vi "Pos ctrl window-Update coord indicators.vi"(9 "Z":sgl, 10 "Y":sgl, 11 "X":sgl) -> ()   [LabVIEW 2020]
uses:
  Globals/Pos ctrl window globals.vi
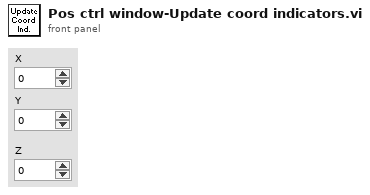
[diagram p1: front panel]
types:
  T1 = typedef "Pos Ctrl window refs cluster.ctl" = cluster{"menu reference":refnum<k9>, "X Coordinate ctrl":refnum<vi>, "Y Coordinate ctrl":refnum<vi>, "Z Coordinate ctrl":refnum<vi>, "Speed setting ctrl":refnum<vi>, "Up":refnum<vi>, "Down":refnum<vi>, "Left":refnum<vi>, "Right":refnum<vi>, "Z move up":refnum<vi>, "Z move down":refnum<vi>, "Down-left":refnum<vi>, "Down-right":refnum<vi>, "Up-left":refnum<vi>, "Up-right":refnum<vi>, "Step = size of image":refnum<vi>, "XY step (um)":refnum<vi>, "Z step (um)":refnum<vi>}
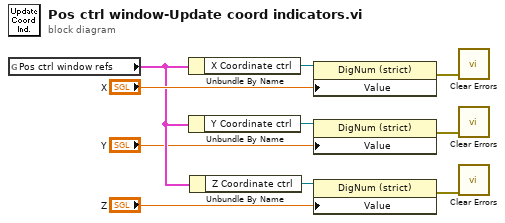
[diagram p0: block diagram]
diagram:
  n1 = global read "Pos ctrl window globals.vi" "Pos ctrl window refs"() -> (w2:T1)
  n2 = Unbundle By Name(w2) -> ("X Coordinate ctrl"=w10:refnum<vi>)
  n3 = Unbundle By Name(w2) -> ("Y Coordinate ctrl"=w3:refnum<vi>)
  n4 = Unbundle By Name(w2) -> ("Z Coordinate ctrl"=w9:refnum<vi>)
  n5 = property on="Property Node" class="DigNum (strict)"(reference=w10, "Value"="X") -> (error out=w8:errorcluster)  [unwired: 1 in, 1 out]
  n6 = property on="Property Node" class="DigNum (strict)"(reference=w3, "Value"="Y") -> (error out=w4:errorcluster)  [unwired: 1 in, 1 out]
  n7 = property on="Property Node" class="DigNum (strict)"(reference=w9, "Value"="Z") -> (error out=w7:errorcluster)  [unwired: 1 in, 1 out]
  n8 = call <vilib>:"Clear Errors.vi"("error in (no error)"=w8) -> ()  [unwired: 5 in, 2 out]
  n9 = call <vilib>:"Clear Errors.vi"("error in (no error)"=w4) -> ()  [unwired: 5 in, 2 out]
  n10 = call <vilib>:"Clear Errors.vi"("error in (no error)"=w7) -> ()  [unwired: 5 in, 2 out]
